vi "2.4.vi"() -> ()   [LabVIEW 2020]
panel:
  out "String":string
  out "C":dbl
  in  "B":dbl
  in  "A":dbl
  in  "Ring":u16(ring) items=["DEFAULT", "SUMAR", "RESTAR", "MULTIPLICAR", "DIVIDIR"]
  # "EL RESULTADO DE LA"
  # "ES"
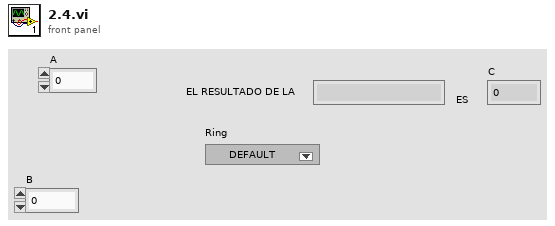
[diagram p1: front panel]
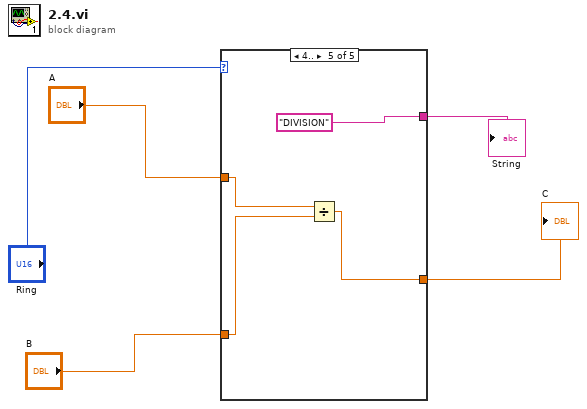
[diagram p0: block diagram]
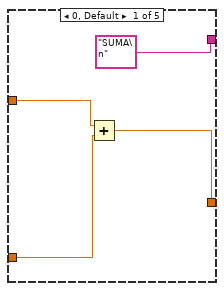
[diagram p2: hidden frame]
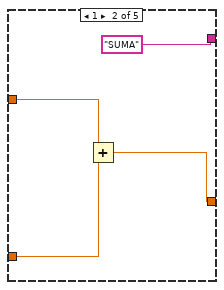
[diagram p3: hidden frame]
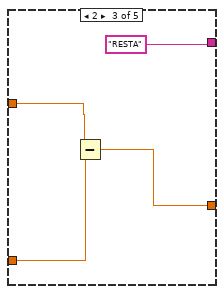
[diagram p4: hidden frame]
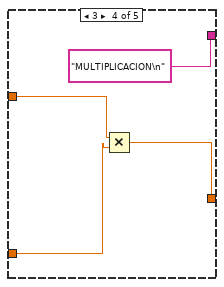
[diagram p5: hidden frame]
diagram:
  n1 = case shown="4.." "Ring" {
    tunnel: "A" -> [w9 w13 w17 w21 w25]
    tunnel: "B" -> [w8 w12 w16 w20 w24]
    tunnel: [w7 w11 w15 w19 w23] -> w3
    tunnel: ["SUMA\n" "SUMA" "RESTA" "MULTIPLICACION\n" "DIVISION"] -> w1
    frame 0, Default {
      n2 = Add(x=w9, y=w8) -> (x+y=w7:dbl)
    }
    frame 1 {
      n3 = Add(x=w13, y=w12) -> (x+y=w11:dbl)
    }
    frame 2 {
      n4 = Subtract(x=w17, y=w16) -> (x-y=w15:dbl)
    }
    frame 3 {
      n5 = Multiply(x=w21, y=w20) -> (x*y=w19:dbl)
    }
    frame 4.. {
      n6 = Divide(x=w25, y=w24) -> (x/y=w23:dbl)
    }
  }
  "C" <- w3
  "String" <- w1
